vi "Init Mixed Mode Command.vi"(2 "error in (no error)":errorcluster) -> (0 "error out":errorcluster, 1 "Command Data":T1)   [LabVIEW 2009]
uses:
  Target Data.ctl
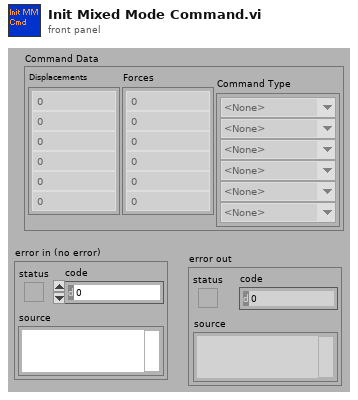
[diagram p1: front panel]
types:
  T1 = typedef "Target Data.ctl" = cluster{"Displacements":dbl[], "Command Type":enum16{"<None>", "Displacement", "Force"}[], "Forces":dbl[]}
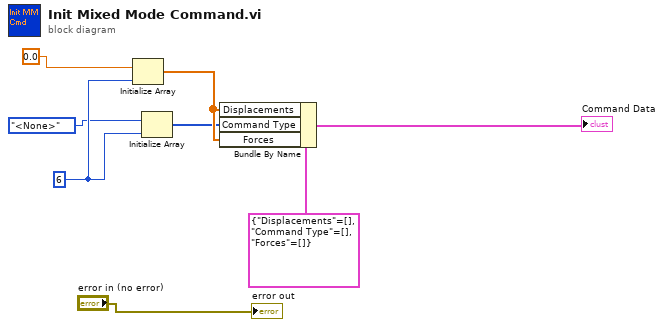
[diagram p0: block diagram]
diagram:
  w6 = 6 ("dimension size")
  n1 = Initialize Array(0.0, w6) -> (w7:dbl[])
  n2 = Initialize Array(enum16{"<None>", "Displacement", "Force"}."<None>" ("Enum"), w6) -> (w4:enum16{"<None>", "Displacement", "Force"}[])
  n3 = Bundle By Name(cluster=T1 {"Displacements"=[], "Command Type"=[], "Forces"=[]} ("Command Data"), "Displacements"=w7, "Command Type"=w4, "Forces"=w7) -> (→"Command Data":T1)
  "error out" <- "error in (no error)"
